vi "FlatToRichnixnet_grpc_ReadStateTimeTriggerResponse.vi"(5 "OutputClusterType":T1, 11 "InputCluster":T3) -> (3 "OutputCluster":T1)   [LabVIEW 2025, in "grpc-xnet_client.lvlib"]
uses:
  grpc-xnet_client.lvlib
  nixnet_grpc_ReadStateTimeTriggerResponse_Flat.ctl
  nixnet_grpc_TimeLocalNetwork_Flat.ctl
  nixnet_grpc_ReadStateTimeTriggerResponse.ctl
  nixnet_grpc_TimeLocalNetwork.ctl
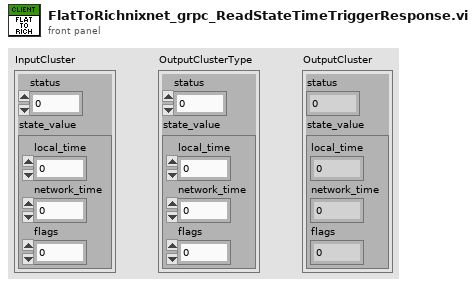
[diagram p1: front panel]
types:
  T1 = typedef "grpc-xnet_client.lvlib/nixnet_grpc_ReadStateTimeTriggerResponse.ctl" = cluster{"status":i32, "state_value":T2}
  T2 = typedef "grpc-xnet_client.lvlib/nixnet_grpc_TimeLocalNetwork.ctl" = cluster{"local_time":u64, "network_time":u64, "flags":u32}
  T3 = typedef "grpc-xnet_client.lvlib/nixnet_grpc_ReadStateTimeTriggerResponse_Flat.ctl" = cluster{"status":i32, "state_value":T4}
  T4 = typedef "grpc-xnet_client.lvlib/nixnet_grpc_TimeLocalNetwork_Flat.ctl" = cluster{"local_time":u64, "network_time":u64, "flags":u32}
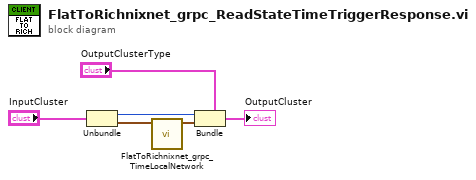
[diagram p0: block diagram]
diagram:
  n1 = Unbundle "Unbundle"("InputCluster") -> ("status"=w3:i32, "state_value"=w2:T4)
  n2 = call "FlatToRichnixnet_grpc_TimeLocalNetwork.vi"("InputCluster"=w2) -> ("OutputCluster"=w1:T2)  [unwired: 10 in]
  n3 = Bundle "Bundle"(cluster="OutputClusterType", "status"=w3, "state_value"=w1) -> (→"OutputCluster":T1)
